vi "On Timeout.vi"(6 "Time":u32, 8 "error in (no error)":errorcluster, 11 "App in":refnum<class "App.lvclass">) -> (0 "error out":errorcluster, 3 "App out":refnum<class "App.lvclass">)   [LabVIEW 2020, in "AR Example.lvlib" / "App.lvclass"]
uses:
  App.lvclass
  App.lvclass/App.ctl
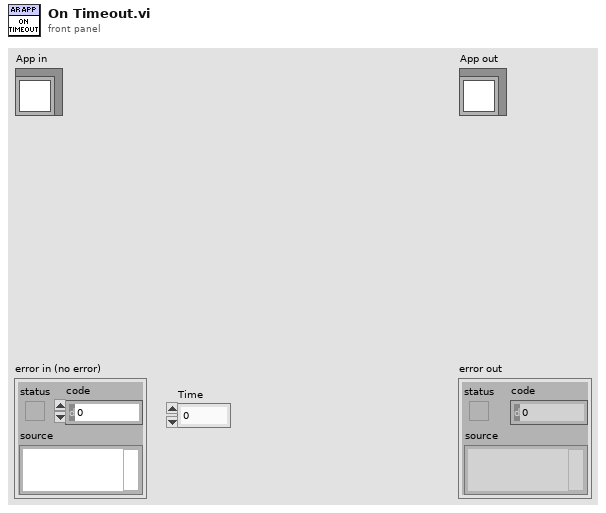
[diagram p1: front panel]
types:
  T1 = typedef "AR Example.lvlib/App.lvclass/Timeout Action.ctl" = enum16{"None", "Setup Camera Action", "Camera Calibration Action"}
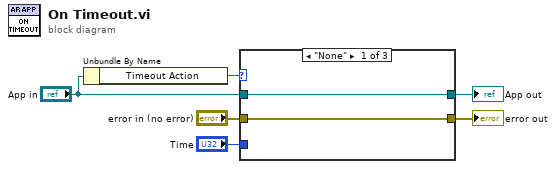
[diagram p0: block diagram]
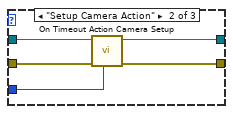
[diagram p2: hidden frame]
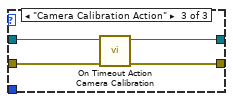
[diagram p3: hidden frame]
diagram:
  n1 = Unbundle By Name("App in") -> ("Timeout Action"=w6:T1)
  n2 = case shown="\"None\"" w6 {
    tunnel: [w7 w11 w15] -> w5
    tunnel: "App in" -> [w7 w12 w16]
    tunnel: [w8 w10 w14] -> w3
    tunnel: "error in (no error)" -> [w8 w13 w17]
    tunnel: "Time" -> [_ w9 _]
    frame "None" {
    }
    frame "Setup Camera Action" {
      n3 = call "On Timeout Action Camera Setup.vi"("Time"=w9, "error in (no error)"=w13, "App in"=w12) -> ("error out"=w10:errorcluster, "App out"=w11:refnum<class "App.lvclass">)  [unwired: 7 in]
    }
    frame "Camera Calibration Action" {
      n4 = call "On Timeout Action Camera Calibration.vi"("error in (no error)"=w17, "App in"=w16) -> ("error out"=w14:errorcluster, "App out"=w15:refnum<class "App.lvclass">)  [unwired: 8 in]
    }
  }
  "error out" <- w3
  "App out" <- w5
